vi "SysInfo-Save Panel Position.vi"(0 "VI Refnum":refnum<vi>, 11 "error in (no error)":errorcluster) -> (15 "error out":errorcluster)   [LabVIEW 2020]
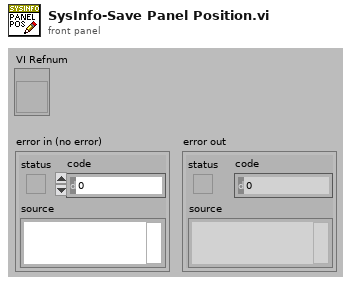
[diagram p1: front panel]
types:
  T1 = typedef "LVRectTypeDef.ctl" = cluster{"Left":i16, "Top":i16, "Right":i16, "Bottom":i16}
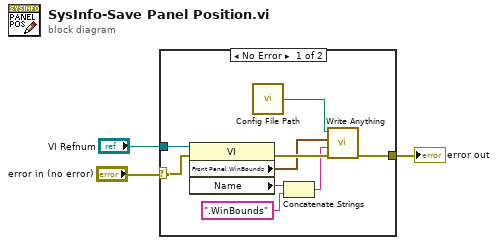
[diagram p0: block diagram]
diagram:
  n1 = case shown="No Error" "error in (no error)" {
    selector: "error in (no error)" -> [w10 w13]
    tunnel: [w7 w13] -> w2
    tunnel: "VI Refnum" -> [w12 _]
    frame No Error {
      n2 = property class="VI"(reference=w12, error in=w10) -> (error out=w9:errorcluster, "Front Panel.WinBounds"=w8:T1, "Name"=w6:string)  [unwired: 1 out]
      n3 = call "Config File Path.vi"() -> ("Default config file name"=w11:path)  [unwired: 1 in]
      n4 = Concatenate Strings(w6, ".WinBounds" ("string")) -> (w5:string)
      n5 = call "Write Anything.vi"("Error In"=w9, "Section Name (Name of \"Anything\")"=w5, "Anything"=w8, "Path (dialog)"=w11) -> ("Error Out"=w7:errorcluster)  [unwired: 6 in, 1 out]
    }
    frame Error {
    }
  }
  "error out" <- w2
